vi "Example.vi"() -> ()   [LabVIEW 2024]
uses:
  U64 Timer Global.vi
panel:
  out "Period":u64
  in  "stop":bool
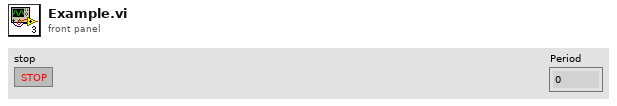
[diagram p1: front panel]
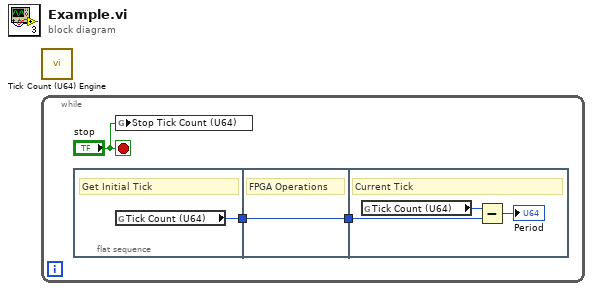
[diagram p0: block diagram]
diagram:
  n1 = call "Tick Count (U64) Engine.vi"() -> ()  [unwired: 12 in]
  n2 = while {
    stop <- "stop" stop-if-true
    n3 = flat-sequence {
      tunnel: [w4] -> w1
      tunnel: [w5] -> w2
      tunnel: w1 -> [w5]
      tunnel: w2 -> [w7]
      frame #0 {
        # "Get Initial Tick"
        n4 = global read "U64 Timer Global.vi" "Tick Count (U64)"() -> (w4:u64)
      }
      frame #1 {
        # "FPGA Operations"
      }
      frame #2 {
        # "Current Tick"
        n5 = global read "U64 Timer Global.vi" "Tick Count (U64)"() -> (w8:u64)
        n6 = Subtract(x=w8, y=w7) -> (x-y=→"Period":u64)
      }
    }
    n7 = global write "U64 Timer Global.vi" "Stop Tick Count (U64)"("stop") -> ()
  }
